vi "Module Extend Initialize.vi"(8 "error in (no error)":errorcluster, 11 "Structure Data":T1) -> (0 "error out":errorcluster, 3 "Event Registration Refnum out":refnum<event-registration>)   [LabVIEW 2020]
uses:
  Def/User_Event.ctl
  DQMH Modules/Module.lvlib
  Def/Main_Data_Package.ctl
  DQMH Modules/Did Init Argument--cluster.ctl
  DQMH Modules/Status Updated Argument--cluster.ctl
  DQMH Modules/Error Reported Argument--cluster.ctl
  DQMH Modules/Stop Argument--cluster.ctl
  DQMH Modules/Get Module Execution Status Argument--cluster.ctl
  DQMH Modules/Broadcast Events--cluster.ctl
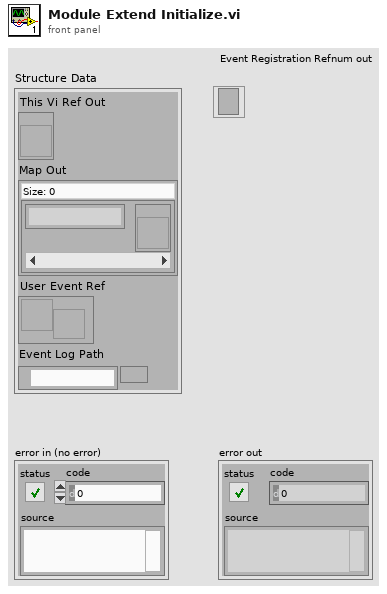
[diagram p1: front panel]
types:
  T1 = typedef "Main_Data_Package.ctl" = cluster{"This Vi Ref Out":refnum<vi>, "Map Out":map{string, refnum<vi>}, "User Event Ref":refnum<user-event>, "Event Log Path":path}
  T2 = typedef "User_Event.ctl" = cluster{"String":string, "Data":variant}
  T3 = enum16{"Initialize", "Get", "Read", "Write", "Release"}
  T4 = typedef "Module.lvlib/Broadcast Events--cluster.ctl" = cluster{"Module Did Init":refnum<user-event>, "Status Updated":refnum<user-event>, "Error Reported":refnum<user-event>, "Module Did Stop":refnum<user-event>, "Update Module Execution Status":refnum<user-event>}
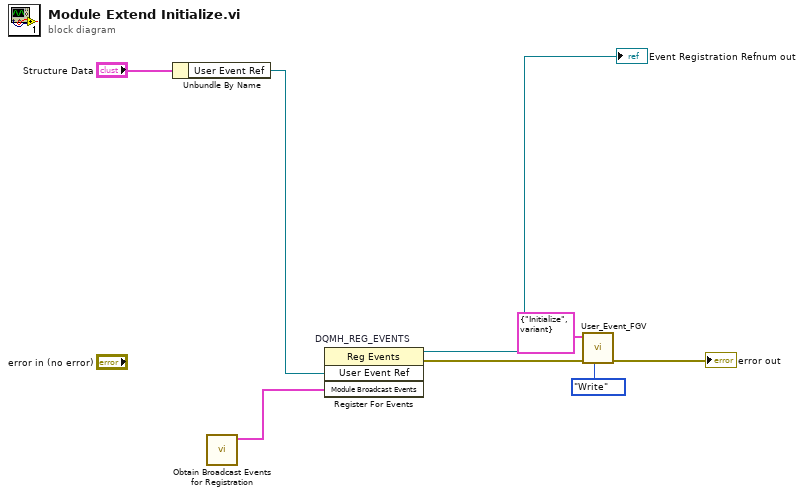
[diagram p0: block diagram]
diagram:
  n1 = Unbundle By Name("Structure Data") -> ("User Event Ref"=w3:refnum<user-event>)
  n2 = call "Obtain Broadcast Events for Registration.vi"() -> ("Module Broadcast Events"=w2:T4)  [unwired: 9 in, 2 out]
  n3 = register-events "DQMH_REG_EVENTS"(w3, w2) -> (reference out=→"Event Registration Refnum out":refnum<event-registration>, error out=w6:errorcluster)  [unwired: 2 in]
  n4 = call "User_Event_FGV.vi"("Method"=T3."Write", "error in"=w6, "User Event"=T2 {"String"="Initialize", "Data"=variant}) -> ("error out"=→"error out":errorcluster)  [unwired: 7 in, 1 out]
